vi "Show Graph SubVi.vi"(1 "Horizontal Segments Parameters":T1(array[cluster]) {"Y rel dist" min=-100.0 max=100.0; "X rel dist" min=-100.0 max=100.0}, 2 "Vertical Segments Parameters":T1(array[cluster]) {"Y rel dist" min=-100.0 max=100.0; "X rel dist" min=-100.0 max=100.0}) -> (0 "Output Array":cluster{"X":dbl, "Y":dbl}[](array[cluster]))   [LabVIEW 2017]
uses:
  Relative Move Enum.ctl
  Show Graph Outter Enum.ctl
  Show Graph Inner Enum.ctl
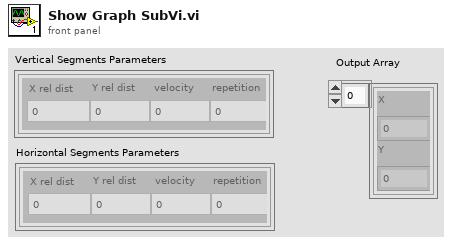
[diagram p1: front panel]
types:
  T1 = cluster{"X rel dist":dbl, "Y rel dist":dbl, "velocity":dbl, "repetition":u32}[]
  T2 = typedef "Relative Move Enum.ctl" = enum16{"Vertical Relative Motion", "Horizontal Relative Motion", "Stop Command"}
  T3 = typedef "Show Graph Outter Enum.ctl" = enum16{"Movment", "Stop Command"}
  T4 = typedef "Show Graph Inner Enum.ctl" = enum16{"Move Y", "Move X", "Stop Command"}
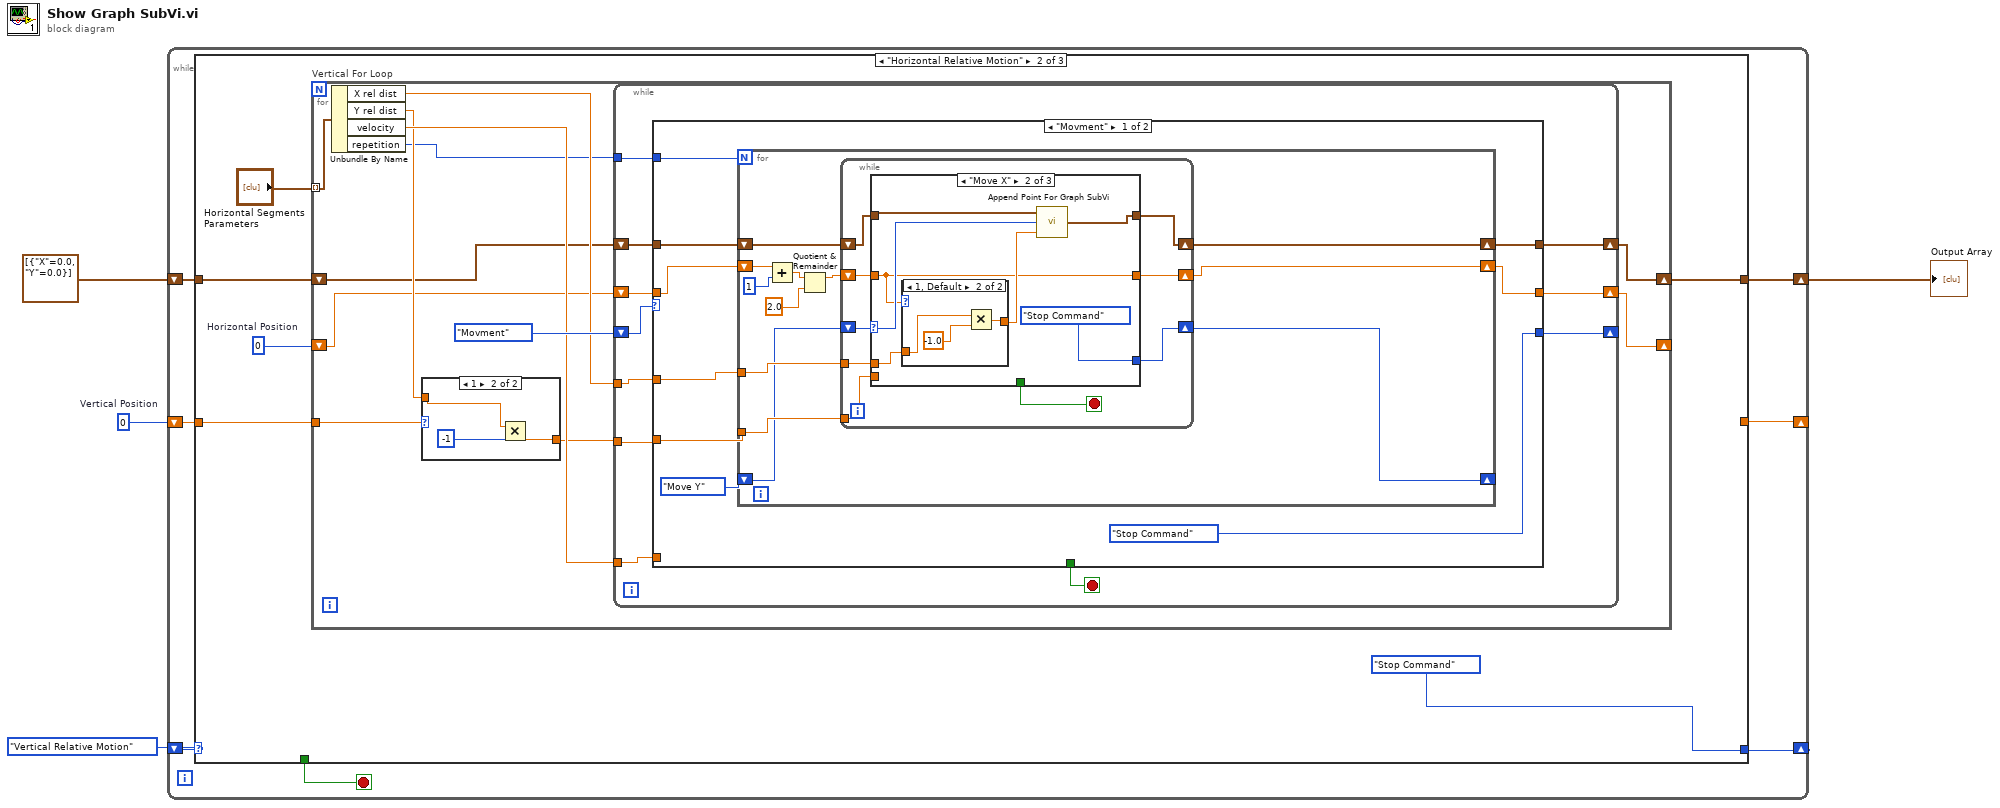
[diagram p0: block diagram]
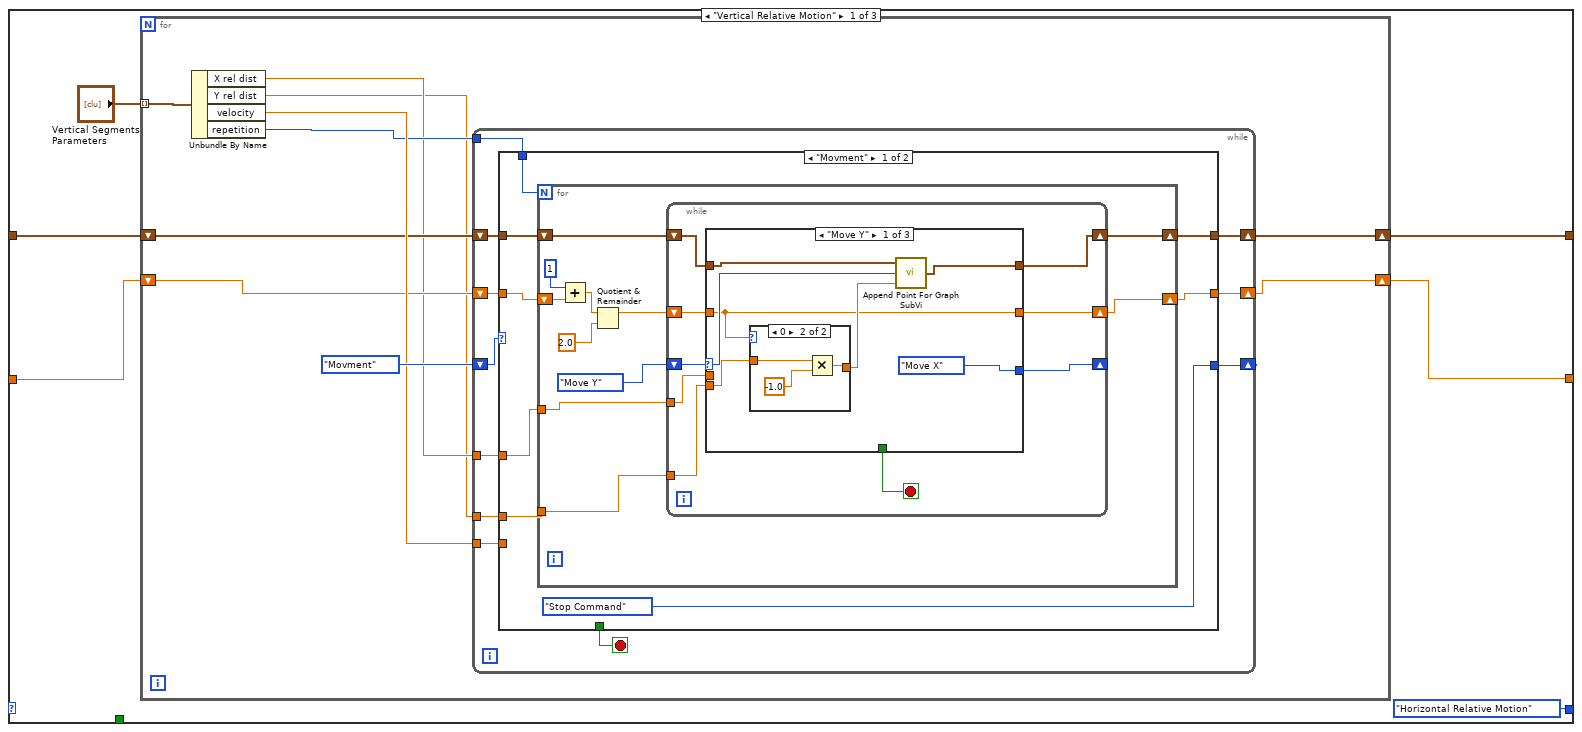
[diagram p2: hidden frame]
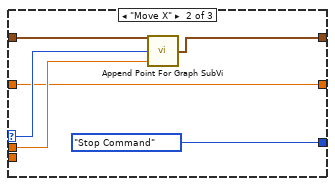
[diagram p4: hidden frame]
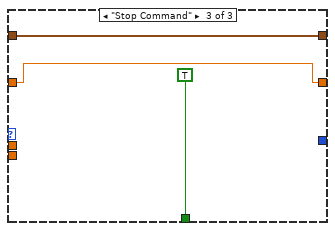
[diagram p5: hidden frame]
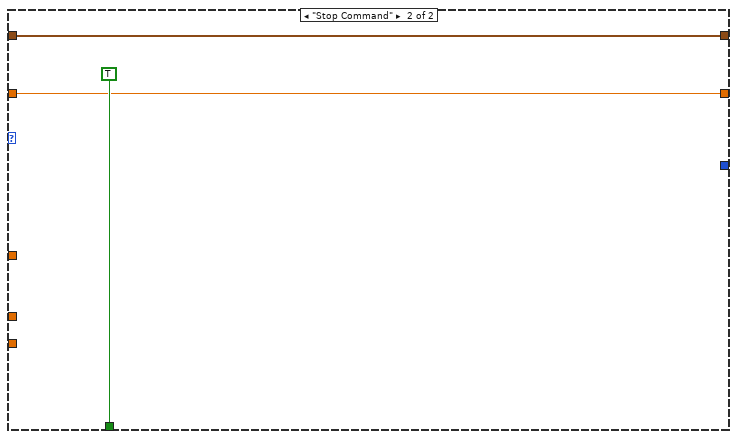
[diagram p6: hidden frame]
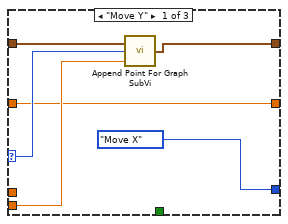
[diagram p7: hidden frame]
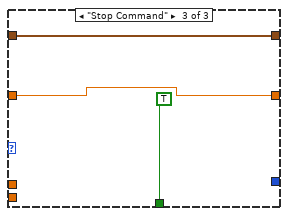
[diagram p9: hidden frame]
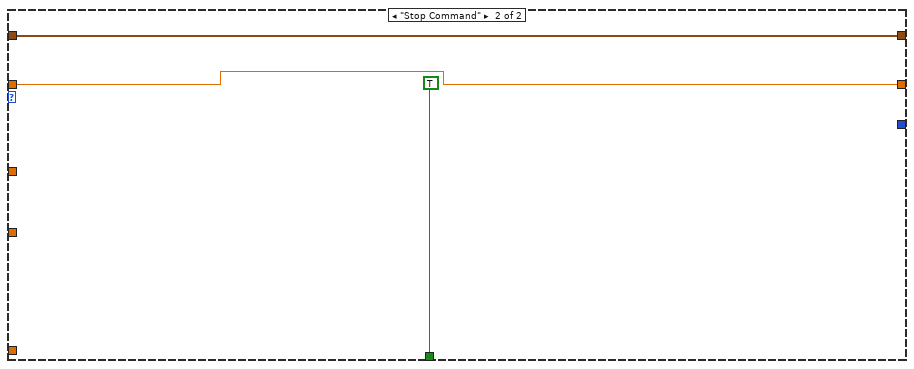
[diagram p10: hidden frame]
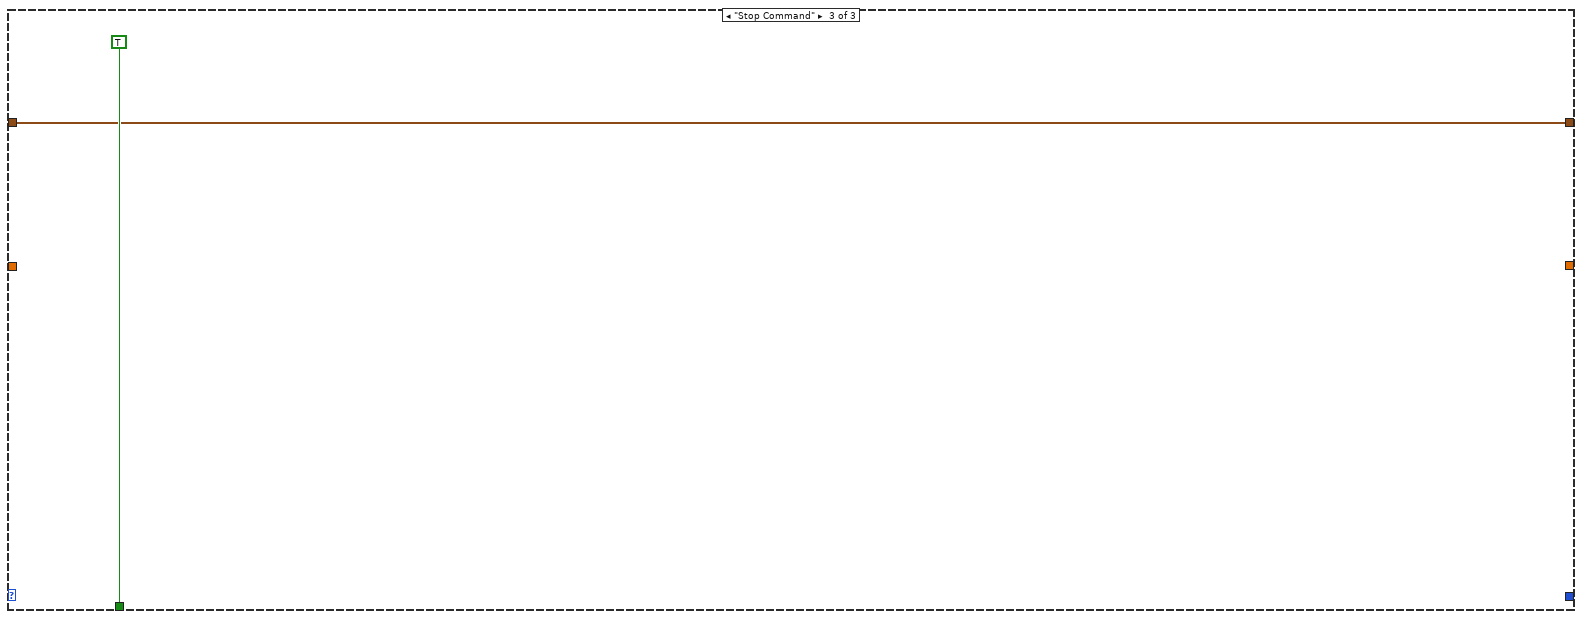
[diagram p12: hidden frame]
diagram:
  w4 = 0  # Vertical Position
  n1 = while {
    shift-right: [w10] -> _
    shift-left: Relative_Move_Enum."Vertical Relative Motion" -> [w11]
    shift-right: [w8] -> _
    shift-left: w4 -> [w9]
    shift-right: [w5] -> w1
    shift-left: cluster{"X":dbl, "Y":dbl}[] [{"X"=0.0, "Y"=0.0}] ("XY Graph") -> [w6]
    stop <- w7 stop-if-true
    n2 = case shown="\"Horizontal Relative Motion\"" w11 {
      tunnel: [Relative_Move_Enum."Horizontal Relative Motion" Relative_Move_Enum."Stop Command" _] -> w10
      tunnel: w9 -> [w12 w91 _]
      tunnel: [w17 _ _] -> w8
      tunnel: [_ _ TRUE] -> w7
      tunnel: w6 -> [w14 w93 w176]
      tunnel: [w13 w92 w176] -> w5
      frame "Vertical Relative Motion" {
        n3 = for {
          tunnel: "Vertical Segments Parameters" -> [w27] mode=indexing
          shift-right: [w18] -> w17
          shift-left: w12 -> [w23]
          shift-right: [w21] -> w13
          shift-left: w14 -> [w22]
          n4 = Unbundle By Name(w27) -> ("X rel dist"=w20:dbl, "Y rel dist"=w19:dbl, "velocity"=w25:dbl, "repetition"=w24:u32)
          n5 = while {
            shift-right: [w36] -> _
            shift-left: Show_Graph_Outter_Enum."Movment" -> [w38]
            tunnel: w24 -> [w35]
            tunnel: w25 -> [w37]
            tunnel: w20 -> [w32]
            tunnel: w19 -> [w33]
            shift-right: [w29] -> w21
            shift-left: w22 -> [w30]
            shift-right: [w28] -> w18
            shift-left: w23 -> [w34]
            stop <- w31 stop-if-true
            n6 = case shown="\"Movment\"" w38 {
              tunnel: w37 -> [_ _]
              tunnel: [Show_Graph_Outter_Enum."Stop Command" _] -> w36
              tunnel: w35 -> [w46 _]
              tunnel: w34 -> [w45 w87]
              tunnel: w33 -> [w44 _]
              tunnel: w32 -> [w40 _]
              tunnel: [_ TRUE] -> w31
              tunnel: w30 -> [w42 w88]
              tunnel: [w41 w88] -> w29
              tunnel: [w39 w87] -> w28
              frame "Movment" {
                n7 = for {
                  N: w46 -> [_]
                  tunnel: w40 -> [w52]
                  tunnel: w44 -> [w53]
                  shift-right: [w49] -> w41
                  shift-left: w42 -> [w50]
                  shift-right: [w48] -> w39
                  shift-left: w45 -> [w54]
                  n8 = Add(x=1, y=w54) -> (x+y=w57:dbl)
                  n9 = Quotient & Remainder(x=w57, y=2.0) -> (x-y*floor(x/y)=w56:dbl)  [unwired: 1 out]
                  n10 = while {
                    shift-right: [w62] -> _
                    shift-left: Show_Graph_Inner_Enum."Move Y" -> [w63]
                    tunnel: w52 -> [w64]
                    tunnel: w53 -> [w65]
                    shift-right: [w59] -> w49
                    shift-left: w50 -> [w60]
                    shift-right: [w58] -> w48
                    shift-left: w56 -> [w66]
                    stop <- w61 stop-if-true
                    n11 = case shown="\"Move Y\"" w63 {
                      selector: w63 -> [w70 w80 _]
                      tunnel: [Show_Graph_Inner_Enum."Move X" Show_Graph_Inner_Enum."Stop Command" _] -> w62
                      tunnel: w66 -> [w67 w78 w84]
                      tunnel: w65 -> [w73 _ _]
                      tunnel: w64 -> [_ w79 _]
                      tunnel: [_ _ TRUE] -> w61
                      tunnel: w60 -> [w71 w82 w85]
                      tunnel: [w68 w81 w85] -> w59
                      tunnel: [w67 w78 w84] -> w58
                      frame "Move Y" {
                        n12 = case shown="0" w67 {
                          tunnel: w73 -> [w74 w75]
                          tunnel: [w74 w76] -> w69
                          frame 1, Default {
                          }
                          frame 0 {
                            n13 = Multiply(x=w75, y=-1.0) -> (x*y=w76:dbl)
                          }
                        }
                        n14 = call "Append Point For Graph SubVi.vi"("Numeric"=w69, "Enum"=w70, "array"=w71) -> ("output array"=w68:cluster{"X Cordinate":dbl, "Y Cordinate":dbl}[])
                      }
                      frame "Move X" {
                        n15 = call "Append Point For Graph SubVi.vi"("Numeric"=w79, "Enum"=w80, "array"=w82) -> ("output array"=w81:cluster{"X Cordinate":dbl, "Y Cordinate":dbl}[])
                      }
                      frame "Stop Command" {
                      }
                    }
                  }
                }
              }
              frame "Stop Command" {
              }
            }
          }
        }
      }
      frame "Horizontal Relative Motion" {
        w90 = 0  # Horizontal Position
        n16 = for "Vertical For Loop" {
          tunnel: "Horizontal Segments Parameters" -> [w107] mode=indexing
          tunnel: w91 -> [w96]
          shift-right: [w99] -> w92
          shift-left: w93 -> [w100]
          shift-right: [w97] -> _
          shift-left: w90 -> [w98]
          n17 = Unbundle By Name(w107) -> ("X rel dist"=w102:dbl, "Y rel dist"=w104:dbl, "velocity"=w105:dbl, "repetition"=w101:u32)
          n18 = case shown="1" w96 {
            tunnel: [w172 w175] -> w103
            tunnel: w104 -> [w172 w173]
            frame 0, Default {
            }
            frame 1 {
              n19 = Multiply(x=w173, y=-1) -> (x*y=w175:dbl)
            }
          }
          n20 = while {
            shift-right: [w116] -> _
            shift-left: Show_Graph_Outter_Enum."Movment" -> [w118]
            tunnel: w105 -> [w117]
            tunnel: w101 -> [w113]
            tunnel: w102 -> [w114]
            tunnel: w103 -> [w115]
            shift-right: [w110] -> w99
            shift-left: w100 -> [w111]
            shift-right: [w108] -> w97
            shift-left: w98 -> [w109]
            stop <- w112 stop-if-true
            n21 = case shown="\"Movment\"" w118 {
              tunnel: w117 -> [_ _]
              tunnel: [Show_Graph_Outter_Enum."Stop Command" _] -> w116
              tunnel: w115 -> [w127 _]
              tunnel: w114 -> [w126 _]
              tunnel: w113 -> [w124 _]
              tunnel: [_ TRUE] -> w112
              tunnel: w111 -> [w122 w170]
              tunnel: [w121 w170] -> w110
              tunnel: w109 -> [w120 w169]
              tunnel: [w119 w169] -> w108
              frame "Movment" {
                n22 = for {
                  N: w124 -> [_]
                  shift-right: [w134] -> _
                  shift-left: Show_Graph_Inner_Enum."Move Y" -> [w135]
                  tunnel: w126 -> [w136]
                  tunnel: w127 -> [w137]
                  shift-right: [w132] -> w121
                  shift-left: w122 -> [w133]
                  shift-right: [w128] -> w119
                  shift-left: w120 -> [w130]
                  n23 = Add(x=w130, y=1) -> (x+y=w131:dbl)
                  n24 = Quotient & Remainder(x=w131, y=2.0) -> (x-y*floor(x/y)=w139:dbl)  [unwired: 1 out]
                  n25 = while {
                    tunnel: w137 -> [w147]
                    tunnel: w136 -> [w146]
                    shift-right: [w144] -> w134
                    shift-left: w135 -> [w145]
                    shift-right: [w141] -> w132
                    shift-left: w133 -> [w142]
                    shift-right: [w140] -> w128
                    shift-left: w139 -> [w148]
                    stop <- w143 stop-if-true
                    n26 = case shown="\"Move X\"" w145 {
                      selector: w145 -> [w151 w157 _]
                      tunnel: [Show_Graph_Inner_Enum."Move X" Show_Graph_Inner_Enum."Stop Command" _] -> w144
                      tunnel: w148 -> [w149 w155 w166]
                      tunnel: w147 -> [w150 _ _]
                      tunnel: w146 -> [_ w160 _]
                      tunnel: [_ _ TRUE] -> w143
                      tunnel: w142 -> [w153 w159 w167]
                      tunnel: [w152 w158 w167] -> w141
                      tunnel: [w149 w155 w166] -> w140
                      frame "Move Y" {
                        n27 = call "Append Point For Graph SubVi.vi"("Numeric"=w150, "Enum"=w151, "array"=w153) -> ("output array"=w152:cluster{"X Cordinate":dbl, "Y Cordinate":dbl}[])
                      }
                      frame "Move X" {
                        n28 = case shown="1, Default" w155 {
                          tunnel: w160 -> [w162 w163]
                          tunnel: [w162 w164] -> w156
                          frame 0 {
                          }
                          frame 1, Default {
                            n29 = Multiply(x=w163, y=-1.0) -> (x*y=w164:dbl)
                          }
                        }
                        n30 = call "Append Point For Graph SubVi.vi"("Numeric"=w156, "Enum"=w157, "array"=w159) -> ("output array"=w158:cluster{"X Cordinate":dbl, "Y Cordinate":dbl}[])
                      }
                      frame "Stop Command" {
                      }
                    }
                  }
                }
              }
              frame "Stop Command" {
              }
            }
          }
        }
      }
      frame "Stop Command" {
      }
    }
  }
  "Output Array" <- w1
